vi "Set Security Level CORE.vi"(8 "error in (no error)":errorcluster, 9 "Set or Clear":T1, 10 "New Level":T2, 11 "Door Alarm in":refnum<class "Door Alarm.lvclass">) -> (0 "error out":errorcluster, 2 "Last Action Performed":string, 3 "Door Alarm out":refnum<class "Door Alarm.lvclass">)   [LabVIEW 2014, in "Door Alarm.lvclass"]
uses:
  Door Alarm.lvclass
  Security System/Security Level.ctl
  Security System/Set or Clear.ctl
  Door Alarm.lvclass/Door Alarm.ctl
  Security System/Security System.lvclass
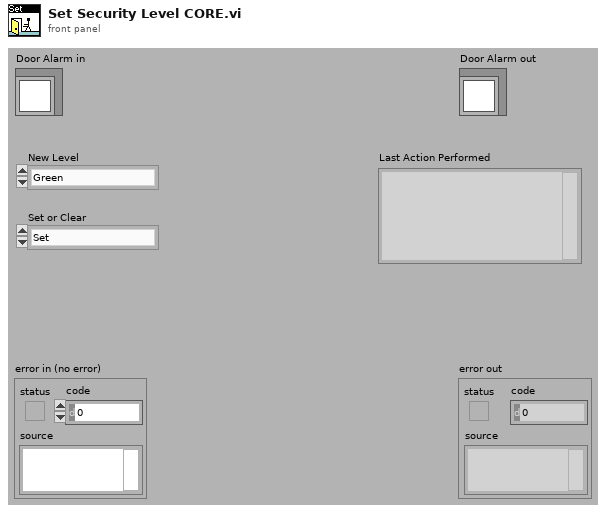
[diagram p1: front panel]
types:
  T1 = typedef "Security System.lvclass/Set or Clear.ctl" = enum16{"Set", "Clear"}
  T2 = typedef "Security System.lvclass/Security Level.ctl" = enum16{"Green", "Yellow", "Orange", "Red"}
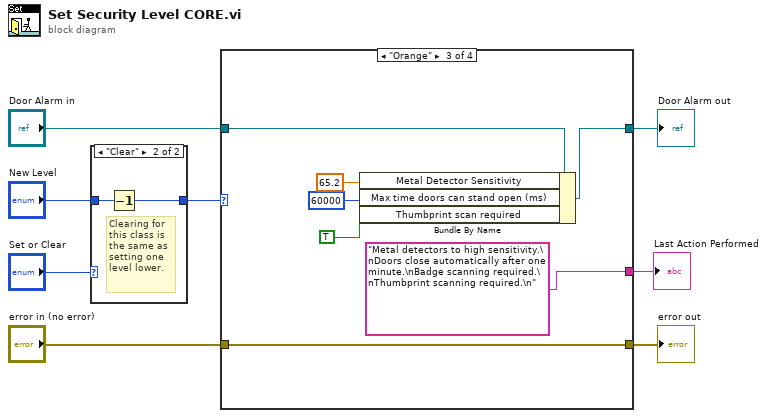
[diagram p0: block diagram]
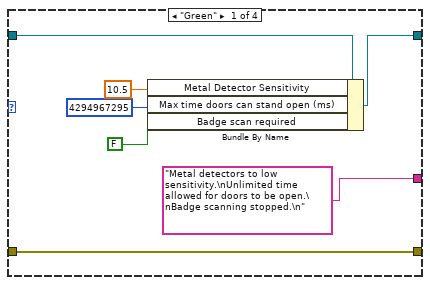
[diagram p3: hidden frame]
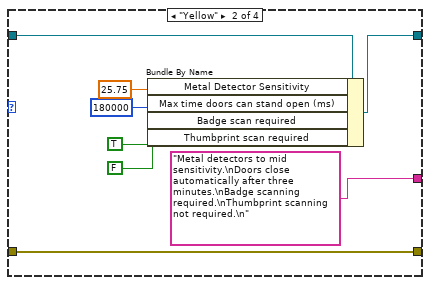
[diagram p4: hidden frame]
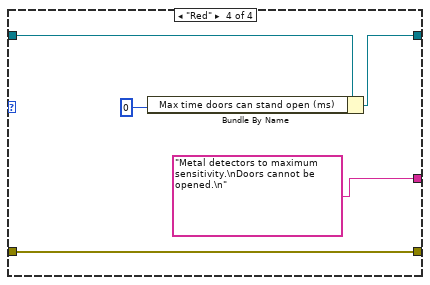
[diagram p5: hidden frame]
diagram:
  n1 = case shown="\"Clear\"" "Set or Clear" {
    tunnel: "New Level" -> [w9 w11]
    tunnel: [w9 w10] -> w2
    frame "Set" {
    }
    frame "Clear" {
      # "Clearing for this class is the same as setting one level lower."
      n2 = Decrement(x=w11) -> (x-1=w10:T2)
    }
  }
  n3 = case shown="\"Orange\"" w2 {
    tunnel: [w13 w21 w28 w35] -> w5
    tunnel: "Door Alarm in" -> [w14 w22 w29 w36]
    tunnel: [w18 w26 w33 w38] -> w7
    tunnel: "error in (no error)" -> [w18 w26 w33 w38]
    tunnel: ["Metal detectors to low sensitivity.\nUnlimited time allowed for doors to be open.\nBadge scanning stopped.\n" ("Last Action Performed") "Metal detectors to mid sensitivity.\nDoors close automatically after three minutes.\nBadge scanning required.\nThumbprint scanning not required.\n" ("Last Action Performed") "Metal detectors to high sensitivity.\nDoors close automatically after one minute.\nBadge scanning required.\nThumbprint scanning required.\n" ("Last Action Performed") "Metal detectors to maximum sensitivity.\nDoors cannot be opened.\n" ("Last Action Performed")] -> w1
    frame "Green" {
      n4 = Bundle By Name(cluster=w14, "Metal Detector Sensitivity"=10.5, "Max time doors can stand open (ms)"=u32 4294967295 ("Door time"), "Badge scan required"=FALSE ("Scan required")) -> (w13:refnum<class "Door Alarm.lvclass">)
    }
    frame "Yellow" {
      n5 = Bundle By Name(cluster=w22, "Metal Detector Sensitivity"=25.75, "Max time doors can stand open (ms)"=u32 180000 ("Door time"), "Badge scan required"=TRUE ("Scan required"), "Thumbprint scan required"=FALSE ("Scan required")) -> (w21:refnum<class "Door Alarm.lvclass">)
    }
    frame "Orange" {
      n6 = Bundle By Name(cluster=w29, "Metal Detector Sensitivity"=65.2, "Max time doors can stand open (ms)"=u32 60000 ("Door time"), "Thumbprint scan required"=TRUE ("Scan required")) -> (w28:refnum<class "Door Alarm.lvclass">)
    }
    frame "Red" {
      n7 = Bundle By Name(cluster=w36, "Max time doors can stand open (ms)"=u32 0 ("Door time")) -> (w35:refnum<class "Door Alarm.lvclass">)
    }
  }
  "error out" <- w7
  "Door Alarm out" <- w5
  "Last Action Performed" <- w1
